vi "set ctp settings.vi"(8 "error in (no error)":errorcluster, 10 "ctp_settings":cluster{"CTPMinError":u32, "CTPFlags":u32}, 11 "id":i32) -> (0 "error out":errorcluster, 3 "function return":i32)   [LabVIEW 2012, in "libximc.lvlib"]
doc: "result_t XIMC_API set_ctp_settings (device_t id, const ctp_settings_t* ctp_settings);"
uses:
  libximc.lvlib
  libximc.dll
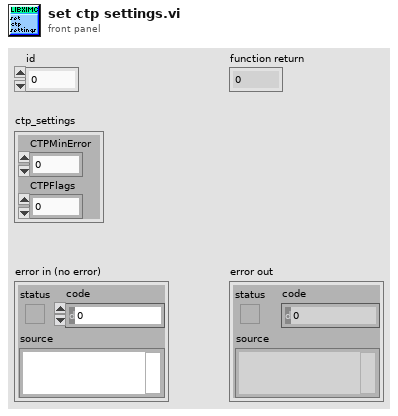
[diagram p1: front panel]
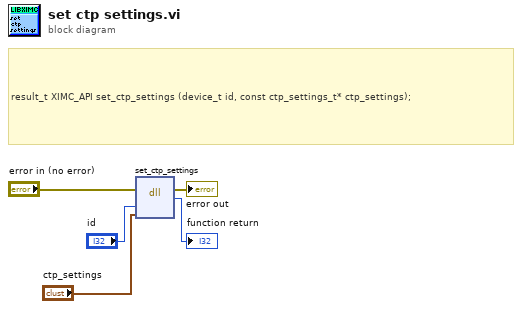
[diagram p0: block diagram]
diagram:
  # "result_t XIMC_API set_ctp_settings (device_t id, const ctp_settings_t* ctp_settings);"
  n1 = dll-call lib="C:/Users/Vasily/Att_examples/LabVIEW_example/libximc.*" fn="set_ctp_settings"(error in="error in (no error)", "id"="id", "ctp_settings"="ctp_settings") -> (error out=→"error out":errorcluster, →"function return":i32)  [unwired: 4 in, 1 out]
